vi "Keithley 24XX Sweep and Acquire Measurements.vi"() -> ()   [LabVIEW 2014]
doc: "Configures a sweep and takes voltage and current readings at each point."
uses:
  Public/Data/Read (Multiple Points).vi
  Keithley 24XX.lvlib
panel:
  out "Status":sgl[](array[numeric])
  out "Resistance":sgl[](array[numeric])
  in  "Source Mode  (0: Voltage)":u16(ring) items=["Voltage", "Current"]
  in  "Serial Configuration":T1={"Baud Rate"=9600, "Parity"=0, "Data Bits"=8, "Stop Bits"=10, "Flow Control"=0} {"Flow Control" items=["None", "XON/XOFF", "RTS/CTS", "XON/XOFF & RTS/CTS", "DTR/DSR", "XON/XOFF & DTR/DSR"]; "Stop Bits" items=["1.0"=10, "1.5"=15, "2.0"=20]; "Data Bits" items=["7"=7, "8"=8]; "Parity" items=["None", "Odd", "Even", "Mark", "Space"]; "Baud Rate" items=["300"=300, "600"=600, "1200"=1200, "2400"=2400, "4800"=4800, "9600"=9600, "19200"=19200]}
  in  "VISA resource name":refnum<visa-resource-name>
  out "Waveform Graph":sgl[][](graph)
  in  "Timeout (10000 ms)":i32=10000 format="%#.6g"
  in  "Maximum Amplitude (2)":dbl=2.0
  in  "Minimum Amplitude (1)":dbl=1.0
  in  "Number of Points (5)":u32=5
  in  "Compliance  Level (0.1)":dbl=0.1
  # "(c) 2006 National Instruments.  ALL RIGHTS RESERVED."
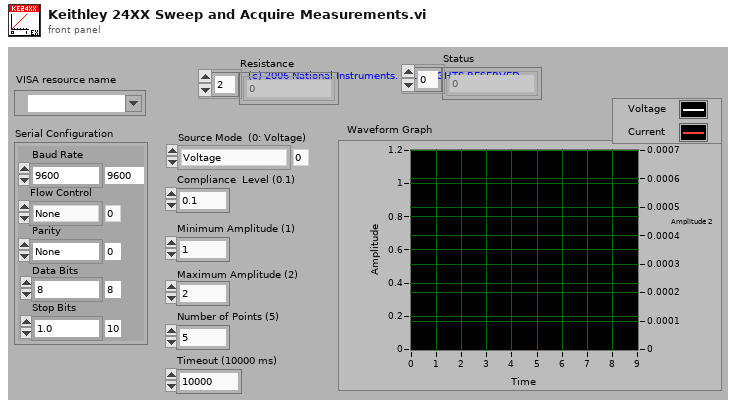
[diagram p1: front panel]
types:
  T1 = cluster{"Baud Rate":u32, "Parity":u16, "Data Bits":u16, "Stop Bits":u16, "Flow Control":u16}
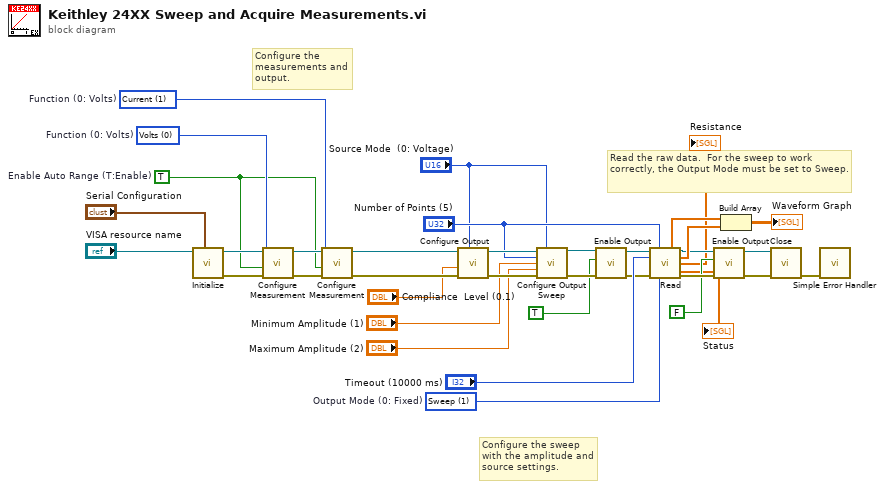
[diagram p0: block diagram]
diagram:
  w5 = TRUE  # Enable Auto Range (T:Enable)
  w6 = u16 1 items=["Volts", "Current", "Resistance"]  # Function (0: Volts)
  w7 = u16 0 items=["Volts", "Current", "Resistance"]  # Function (0: Volts)
  w19 = u16 1 items=["Fixed", "Sweep", "List"]  # Output Mode (0: Fixed)
  # "Read the raw data.  For the sweep to work correctly, the Output Mode must be set to Sweep."
  # "Configure the sweep with the amplitude and source settings."
  # "Configure the measurements and output."
  n1 = call "Initialize.vi"("Serial Configuration"="Serial Configuration", "VISA resource name"="VISA resource name") -> ("error out"=w35:errorcluster, "VISA resource name out"=w36:refnum<visa-resource-name>)  [unwired: 8 in]
  n2 = call "Configure Measurement.vi"("error in (no error)"=w35, "Enable Auto Range (T:Enable)"=w5, "Function (0: Volts)"=w7, "VISA resource name"=w36) -> ("error out"=w34:errorcluster, "VISA resource name out"=w33:refnum<visa-resource-name>)  [unwired: 6 in]
  n3 = call "Configure Measurement.vi"("error in (no error)"=w34, "Enable Auto Range (T:Enable)"=w5, "Function (0: Volts)"=w6, "VISA resource name"=w33) -> ("error out"=w31:errorcluster, "VISA resource name out"=w32:refnum<visa-resource-name>)  [unwired: 6 in]
  n4 = call "Configure Output.vi"("Source Mode  (0: Voltage)"="Source Mode  (0: Voltage)", "error in (no error)"=w31, "Compliance  Level (0.1)"="Compliance  Level (0.1)", "VISA resource name"=w32) -> ("error out"=w30:errorcluster, "VISA resource name out"=w29:refnum<visa-resource-name>)  [unwired: 6 in]
  n5 = call "Configure Output Sweep.vi"("VISA resource name"=w29, "Source Mode  (0: Voltage)"="Source Mode  (0: Voltage)", "Number of Points (5)"="Number of Points (5)", "Minimum Amplitude (1)"="Minimum Amplitude (1)", "Maximum Amplitude (2)"="Maximum Amplitude (2)", "error in (no error)"=w30) -> ("VISA resource name out"=w10:refnum<visa-resource-name>, "error out"=w9:errorcluster)  [unwired: 8 in]
  n6 = call "Enable Output.vi"("error in (no error)"=w9, "Enable Output (T: Enable)"=TRUE, "VISA resource name"=w10) -> ("error out"=w12:errorcluster, "VISA resource name out"=w11:refnum<visa-resource-name>)  [unwired: 7 in]
  n7 = call-poly "Read.vi"("VISA resource name"=w11, "Sample Count (1)"="Number of Points (5)", "Timeout (10000 ms)"="Timeout (10000 ms)", "error in (no error)"=w12, "Output Mode (0: Fixed)"=w19) -> ("Voltage"=w24:sgl[], "VISA resource name out"=w14:refnum<visa-resource-name>, "Current"=w23:sgl[], "Resistance"=→"Resistance":sgl[], "Status"=→"Status":sgl[], "error out"=w15:errorcluster)  [unwired: 4 in, 1 out]
  n8 = call "Enable Output.vi"("error in (no error)"=w15, "Enable Output (T: Enable)"=FALSE, "VISA resource name"=w14) -> ("error out"=w16:errorcluster, "VISA resource name out"=w17:refnum<visa-resource-name>)  [unwired: 7 in]
  n9 = Build Array(w24, w23) -> (→"Waveform Graph":sgl[][])
  n10 = call "Close.vi"("error in (no error)"=w16, "VISA resource name"=w17) -> ("error out"=w18:errorcluster)  [unwired: 9 in]
  n11 = call <vilib>:"Simple Error Handler.vi"("error in (no error)"=w18) -> ()  [unwired: 4 in, 5 out]
